vi "字符串替换.vi"() -> ()   [LabVIEW 2018]
panel:
  in  "停止":bool
  out "替换后偏移量":i32
  out "替换数量":i32
  in  "偏移量(0)":i32
  out "结果字符串":string
  in  "替换字符串":string
  in  "搜索字符串":string
  in  "输入字符串":string
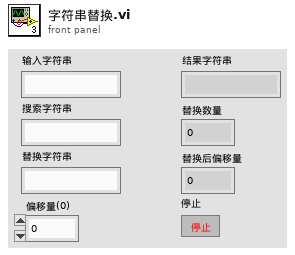
[diagram p1: front panel]
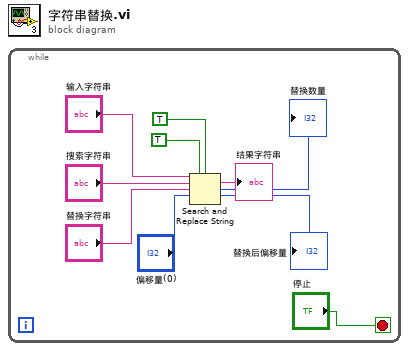
[diagram p0: block diagram]
diagram:
  n1 = while {
    stop <- "停止" stop-if-true
    n2 = Search and Replace String(replace all?=TRUE ("替换全部？(F)"), case sensitive?=TRUE ("忽略大小写？(F)"), input string="输入字符串", search string="搜索字符串", replace string="替换字符串", offset="偏移量(0)") -> (result string=→"结果字符串":string, number of replacements=→"替换数量":i32, offset past replacement=→"替换后偏移量":i32)  [unwired: 2 in, 1 out]
  }
